vi "Measurement UI.vi"() -> ()   [LabVIEW 2021, in "Efficiency_Class D Amplifier_UI.lvlib"]
uses:
  Efficiency_Class D Amplifier_UI.lvlib
  shared/controls/units - snr.ctl
  shared/controls/units - ratio.ctl
  shared/controls/digital output level units.ctl
  shared/ui/controls/view.ctl
  shared/controls/power measurement method.ctl
  UI State.ctl
  <vilib>/Utility/miscctls.llb/LVBoundsTypeDef.ctl
  <vilib>/Utility/miscctls.llb/LVPoint32TypeDef.ctl
  shared/ui/UI Helpers.lvlib
  shared/controls/audio controls.lvlib
panel:
  in  "view legend":T1
  out "time domain":waveform(dbl)[](graph)
  out "frequency domain":cluster{"x0":dbl, "dx":dbl, "magnitude":dbl[]}[](graph)
  out "efficiency (%)":dbl caption="Efficiency" format="%#.2g%"
  out "power loss (W)":dbl caption="Power Loss" format="%#.2g W"
  out "total output power (W)":dbl caption="Total Output Power" format="%#.2g W"
  out "input power (W)":dbl caption="Input Power" format="%#.2g W"
  out "meas table":string[][](table)
  in  "power measurement resource":string="PXI1Slot4/ai0"
  out "output power (W)":dbl[](array[numeric])
  out "SFDR (dBc)":dbl[](array[numeric])
  out "gain":dbl[](array[numeric])
  out "dynamic range (dB)":dbl[](array[numeric])
  out "THD":dbl[](array[numeric])
  out "THD+N":dbl[](array[numeric])
  out "SNR":dbl[](array[numeric])
  out "phase (deg)":dbl[](array[numeric])
  out "amplitude (dBFS)":dbl[](array[numeric])
  out "amplitude (Vrms)":dbl[](array[numeric])
  out "frequency (Hz)":dbl[](array[numeric])
  out "channel names":string[](array[string])
  in  "Configuration tab":enum32{"Protocol", "Measurement", "Units"}(tab)
  in  "enable dither":bool caption="Enable dither"
  in  "master clock channel list":string caption="Master Clock Channel"
  in  "digital channel list":string caption="Digital Audio Channel"
  in  "logic level":enum32{"3.3 V", "1.8 V", "1.2 V"}(ring) caption="Logic level"
  in  "master clock rate":dbl=12288000.0 caption="Master clock rate" format="%#_6pHz"
  out "Bit clock rate":dbl=3072000.0 format="%#_6pHz"
  in  "number of channels":u32=2 caption="Number of channels"
  in  "TDM":bool
  in  "RJ":bool
  in  "LJ":bool
  in  "I2S":bool
  in  "bit clock edge sync":enum32{"Rising", "Falling"}(ring)=enum."Falling" caption="Bit clock edge sync"
  in  "frame clock rate":dbl=48000.0 caption="Frame clock rate" format="%#_6pHz"
  in  "data justification":enum32{"Left Justified", "Right Justified"}(ring) caption="Data justification"
  in  "endianness":enum32{"MSB First", "LSB First"}(ring) caption="Endianness"
  in  "bit depth":u32=24 caption="Bit depth"
  in  "channel length":u32=32 caption="Channel length"
  in  "frame sync edge for channel 0":enum32{"Rising", "Falling"}(ring)=enum."Falling" caption="Frame sync edge for Channel 0"
  in  "sense resistor (Ohms)":dbl caption="Sense Resistor" format="%#_g Ohms"
  in  "power supply current limit":dbl caption="Current Limit" format="%#_g A"
  in  "power supply voltage":dbl caption="Power Supply Voltage" format="%#_g V"
  in  "power meas resource":refnum<k15> caption="Resource"
  in  "power measurement method":T2 caption="Method"
  in  "output level":dbl=-1.0 caption="Output level" format="%#_3f"
  in  "output level units":T3
  in  "min settling cycles":u32 caption="Minimum settling cycles"
  in  "min settling time (s)":dbl=0.1 caption="Minimum settling time" format="%#_6ps"
  in  "min measurement cycles":u32 caption="Minimum measurement cycles"
  in  "min measurement time (s)":dbl=0.1 caption="Minimum measurement time" format="%#_6ps"
  in  "Acquisition channel":tag
  in  "acq sampling rate":dbl=51200.0 caption="Sample rate" format="%#.6pHz"
  in  "lowpass filter":T4(ring) caption="Lowpass filter"
  in  "highpass filter":enum32{"DC", "AC"}(ring) caption="Highpass filter"
  in  "band start":dbl=20.0 caption="Band start" format="%#_6pHz"
  in  "band stop":dbl=20000.0 caption="Band stop" format="%#_6pHz"
  in  "weighting filter":T5(ring)=enum."A-weighting" caption="Weighting filter"
  in  "load impedance":dbl=4.0 caption="Load impedance" format="%#_6p Ohms"
  in  "output range (pk-pk)":dbl=15.0 caption="Output range" format="%.3p Vpk-pk"
  in  "signal frequency":dbl=1000.0 caption="Frequency" format="%#_6pHz"
  in  "gain units":T6 caption="Gain"
  in  "THD units":T6 caption="THD"
  in  "THD+N units":T6 caption="THD+N"
  in  "SNR units":T7 caption="SNR"
  in  "channel 0 offset":u32=1
  out "fft - data":dbl[](array[numeric])
  out "fft - df":dbl
  out "fft - f0":dbl
  out "wfm - data":dbl[](array[numeric])
  out "wfm - dt":dbl
  out "wfm - t0":dbl
  in  "acq channel":string="PXI1Slot4/ai0"
  in  "signal phase":dbl caption="phase"
  # "hidden controls - used to sync with MeasLink"
  # "hidden indicators"
  # "Protocols"
  # "Audio Protocol"
  # "Clock Settings"
  # "Signal Level"
  # "Harware Resource"
  # "Filters"
  # "Output"
  # "Acquisition"
  # "Power"
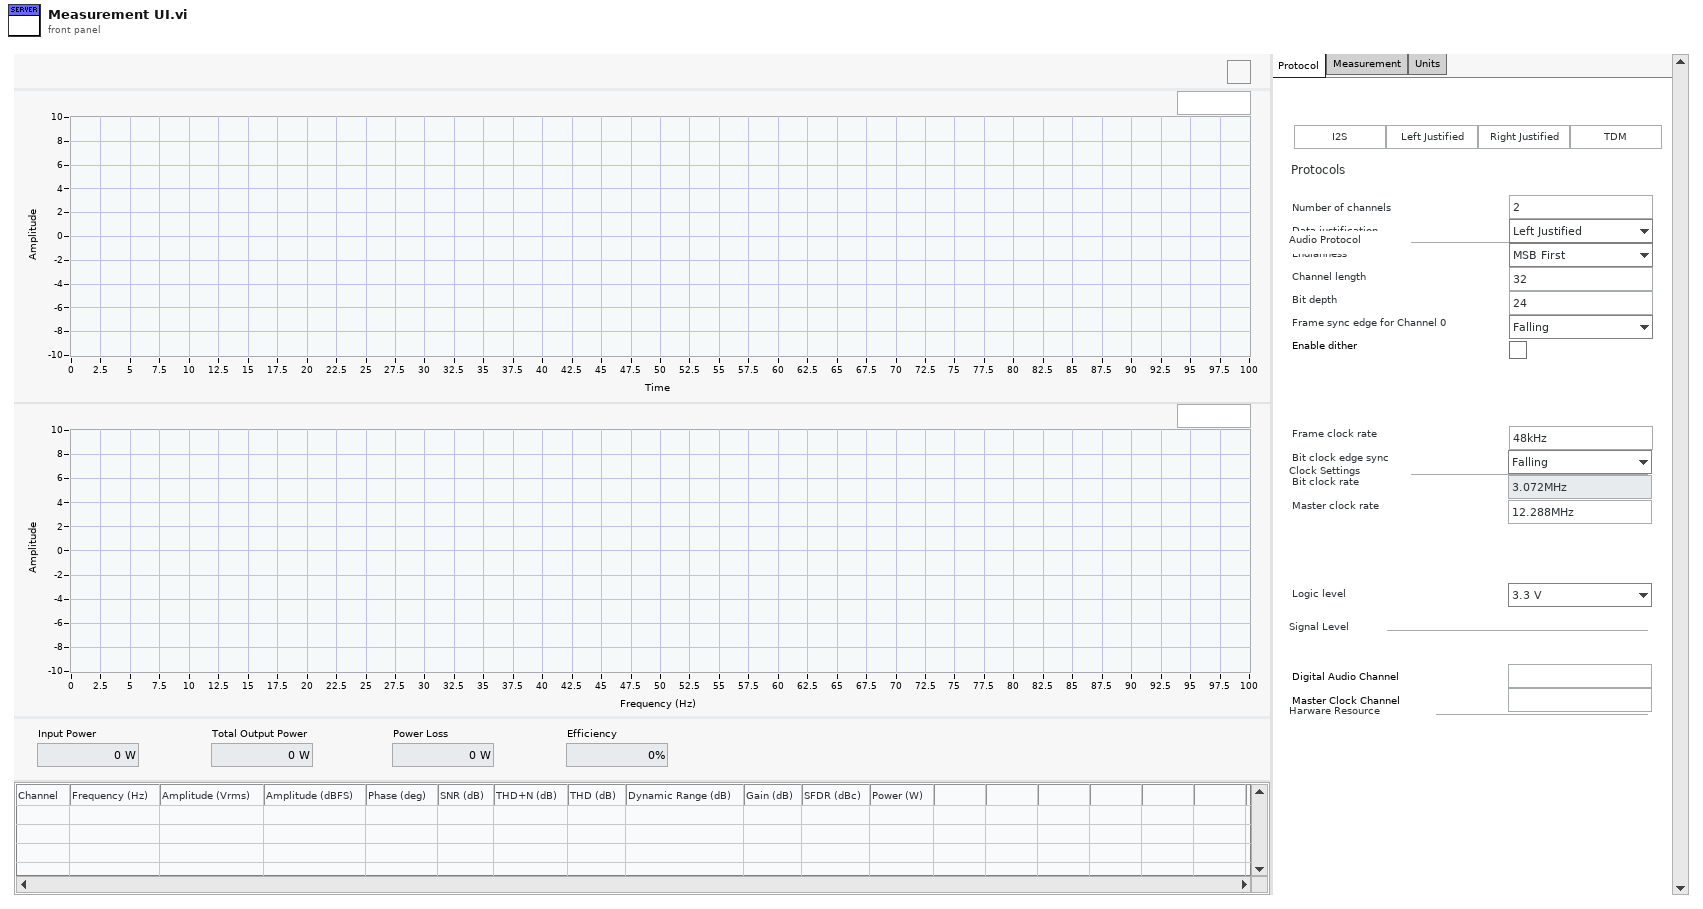
[diagram p1: front panel]
types:
  T1 = typedef "UI Helpers.lvlib/view.ctl" = bool
  T2 = typedef "power measurement method.ctl" = enum32{"SMU", "DMM"}
  T3 = typedef "audio controls.lvlib/digital output level units.ctl" = enum32{"% FS", "dBFS"}
  T4 = enum32{"No filter", "AES17 20kHz", "AES17 40kHz"}
  T5 = enum32{"Linear", "A-weighting", "B-weighting", "C-weighting"}
  T6 = typedef "audio controls.lvlib/units - ratio.ctl" = enum32{"dB", "%", "x/y"}
  T7 = typedef "audio controls.lvlib/units - snr.ctl" = enum32{"dB", "x/y"}
  T8 = typedef "Efficiency_Class D Amplifier_UI.lvlib/UI State.ctl" = cluster{"Graph Size":T9, "Legend Visible":bool, "Mouse Coords":T10}
  T9 = typedef "LVBoundsTypeDef.ctl" = cluster{"Width":u32, "Height":u32}
  T10 = typedef "LVPoint32TypeDef.ctl" = cluster{"Horizontal":i32, "Vertical":i32}
  T11 = typedef "LVPointTypeDef.ctl" = cluster{"Horizontal":i16, "Vertical":i16}
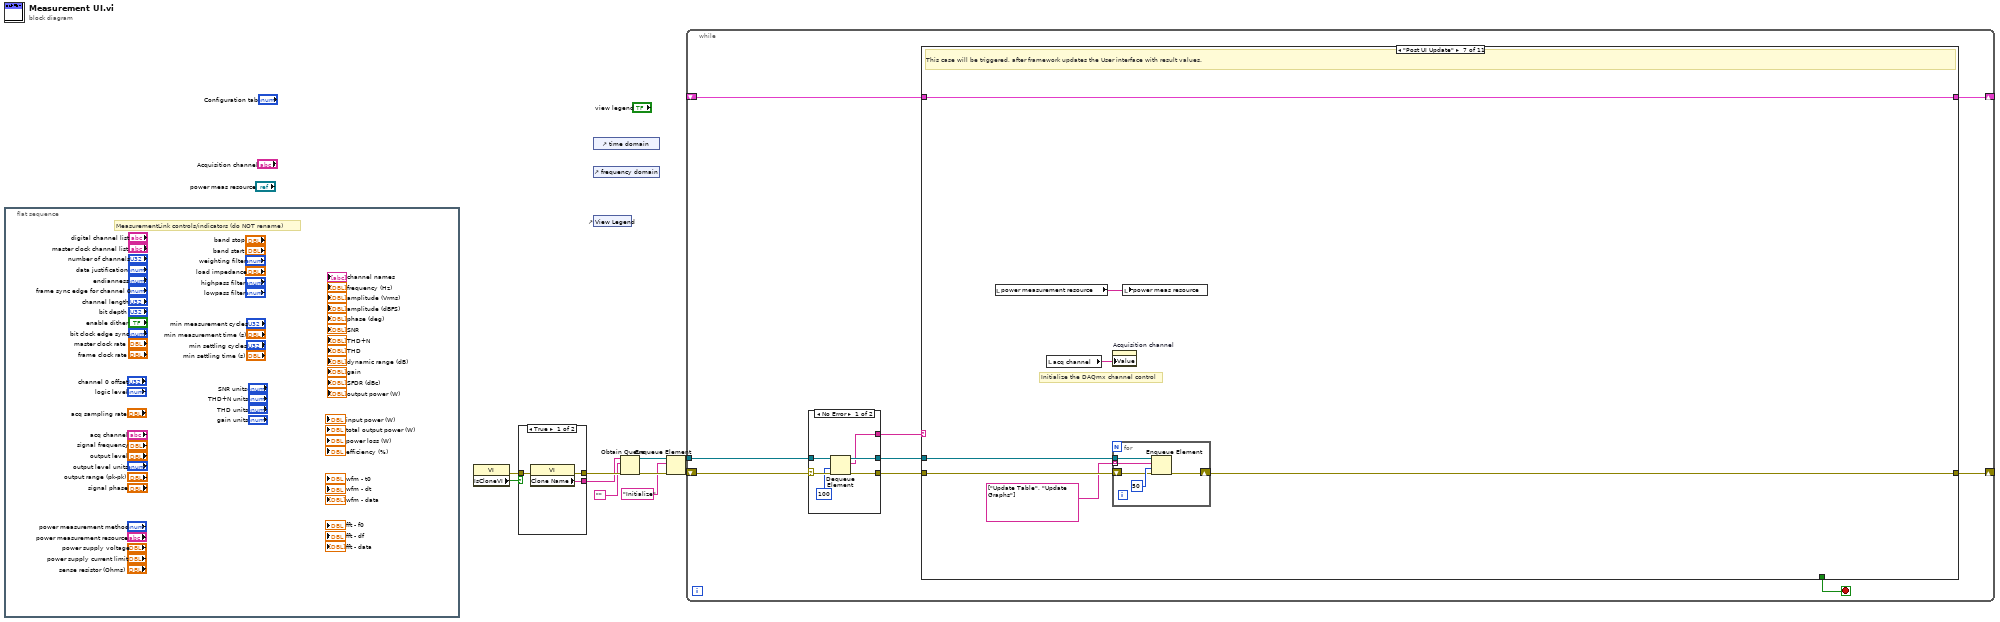
[diagram p0: block diagram]
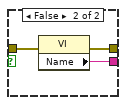
[diagram p2: hidden frame]
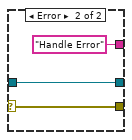
[diagram p3: hidden frame]
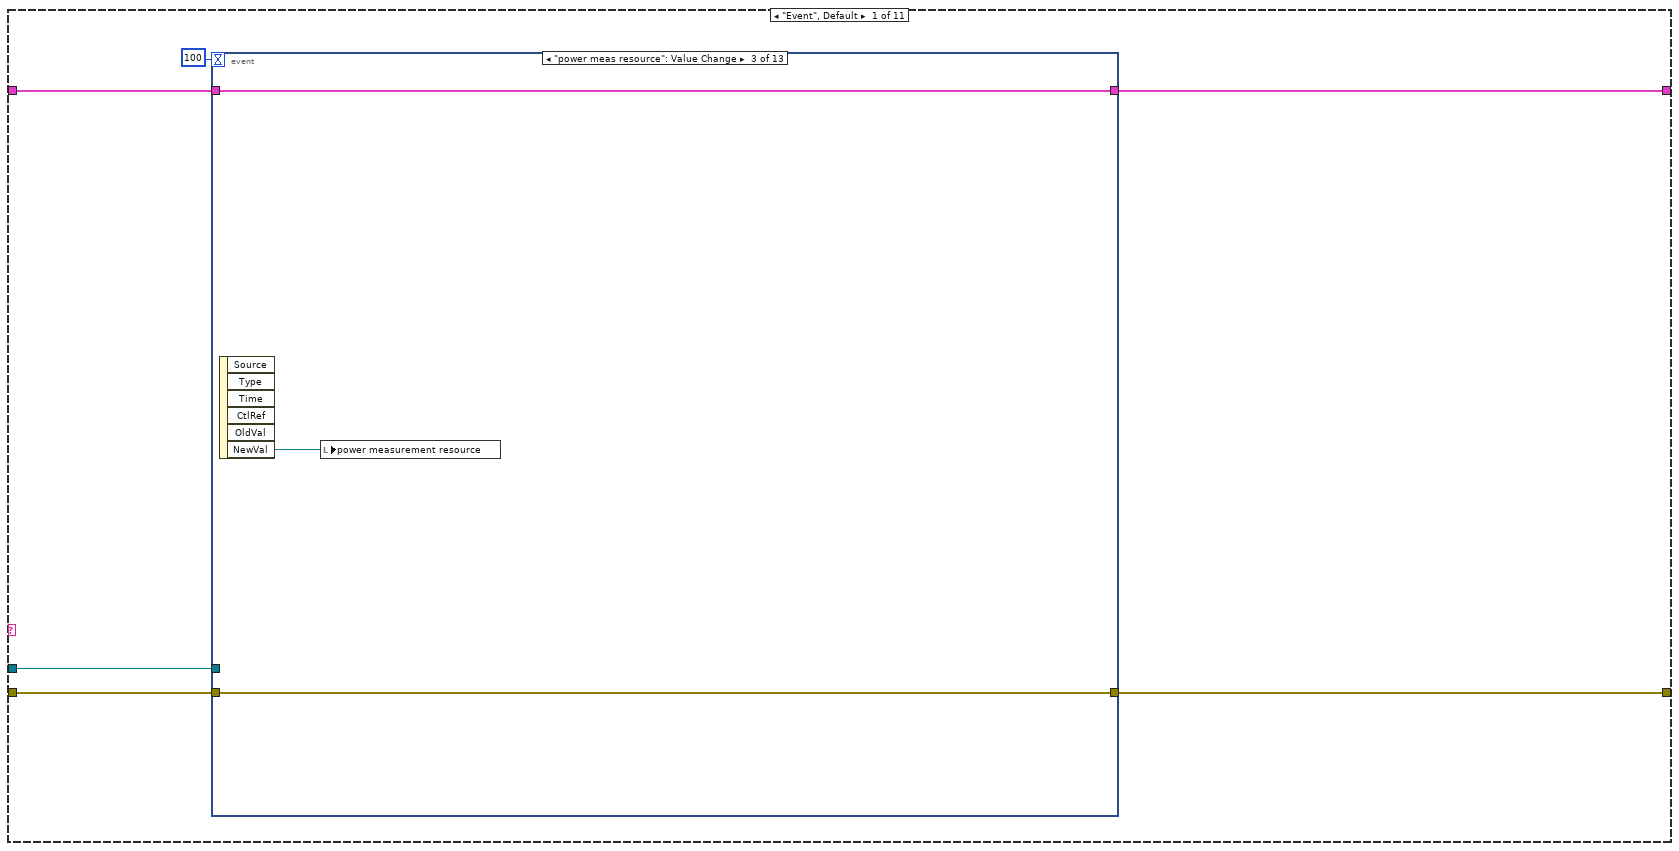
[diagram p4: hidden frame]
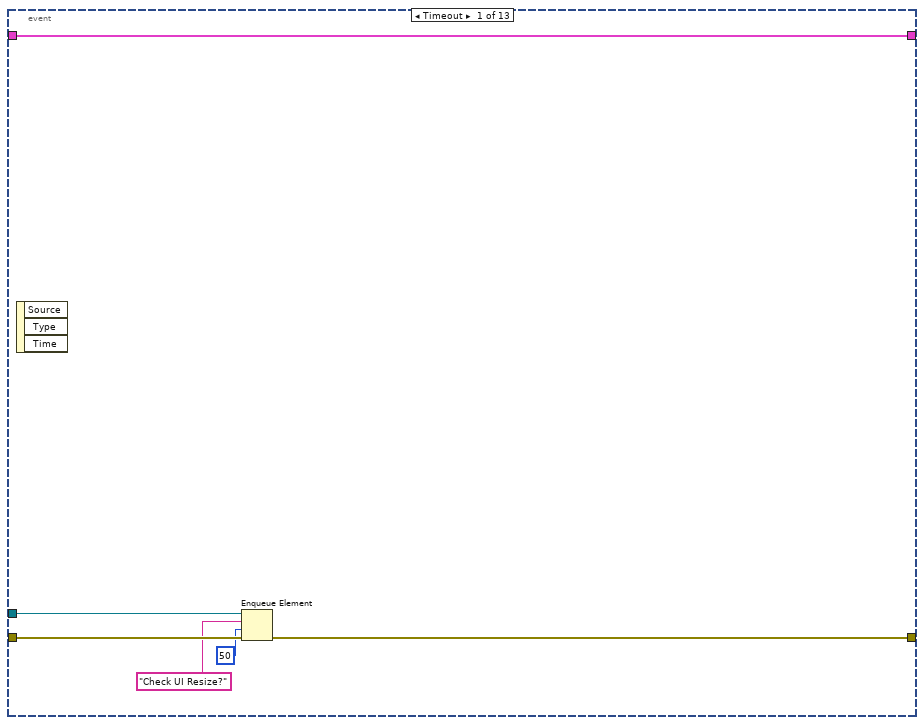
[diagram p5: hidden frame]
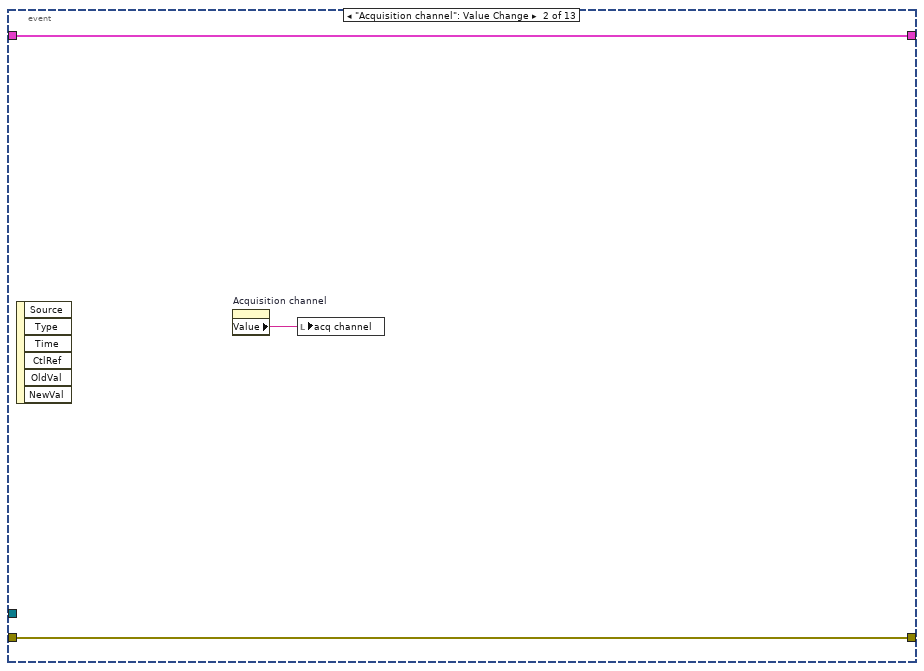
[diagram p6: hidden frame]
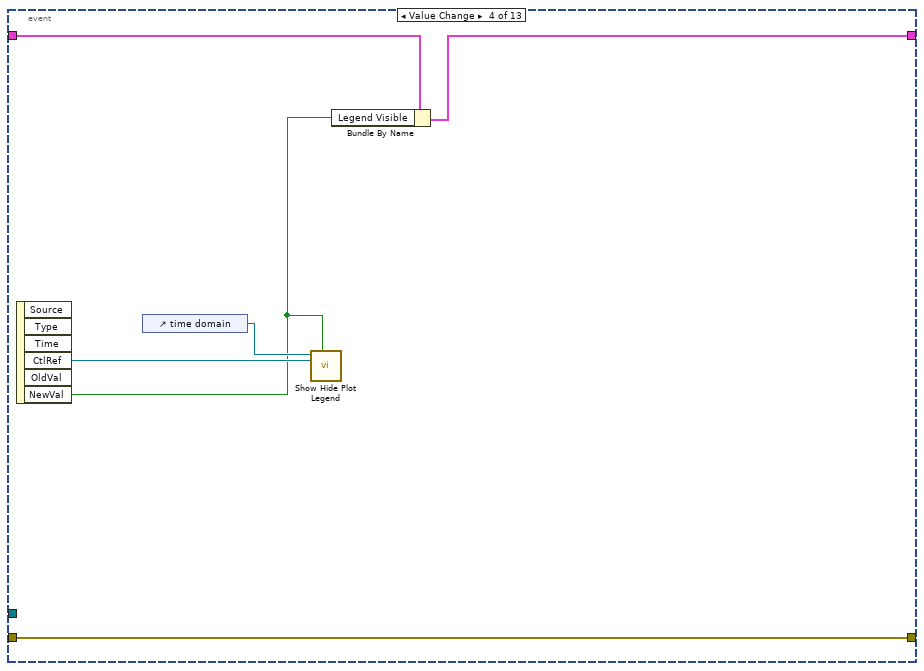
[diagram p7: hidden frame]
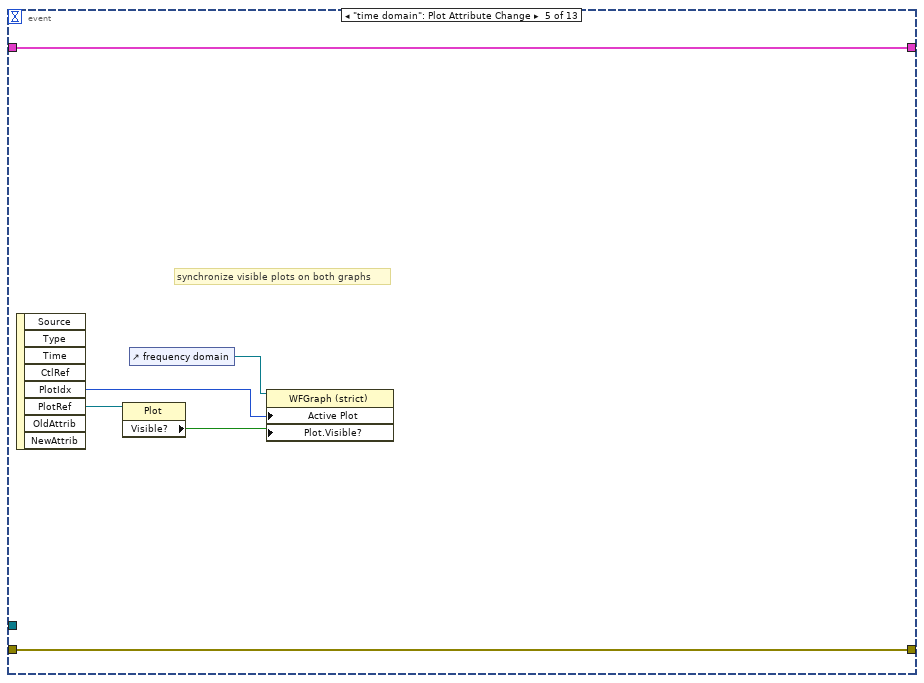
[diagram p8: hidden frame]
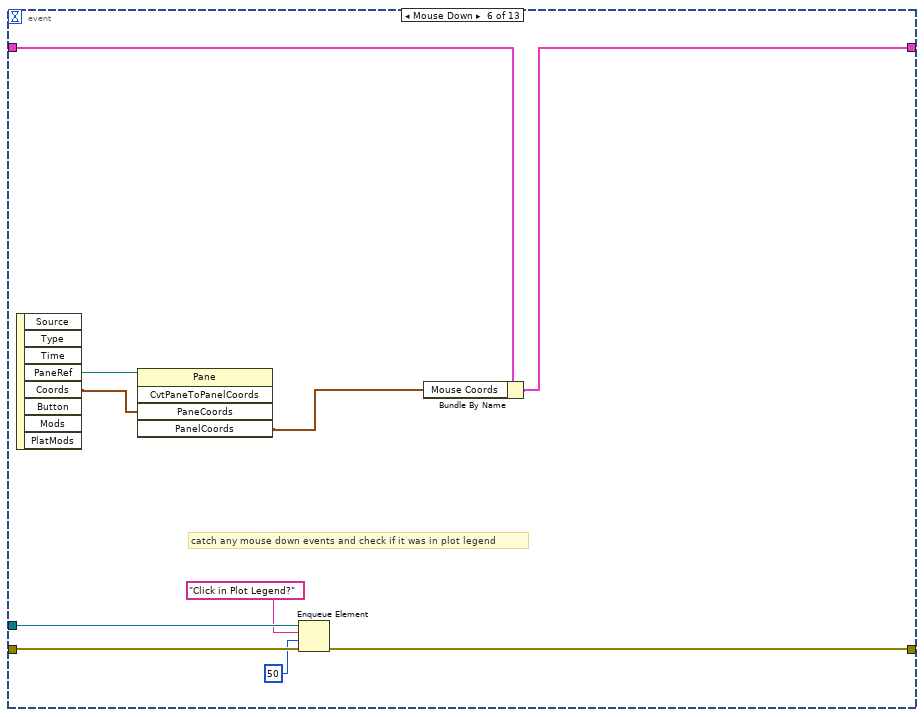
[diagram p9: hidden frame]
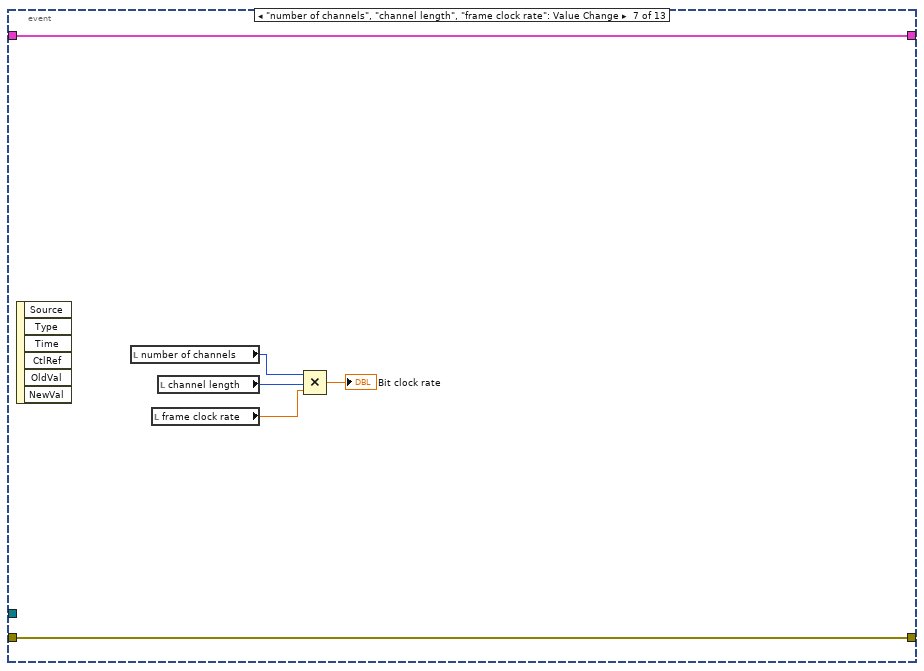
[diagram p10: hidden frame]
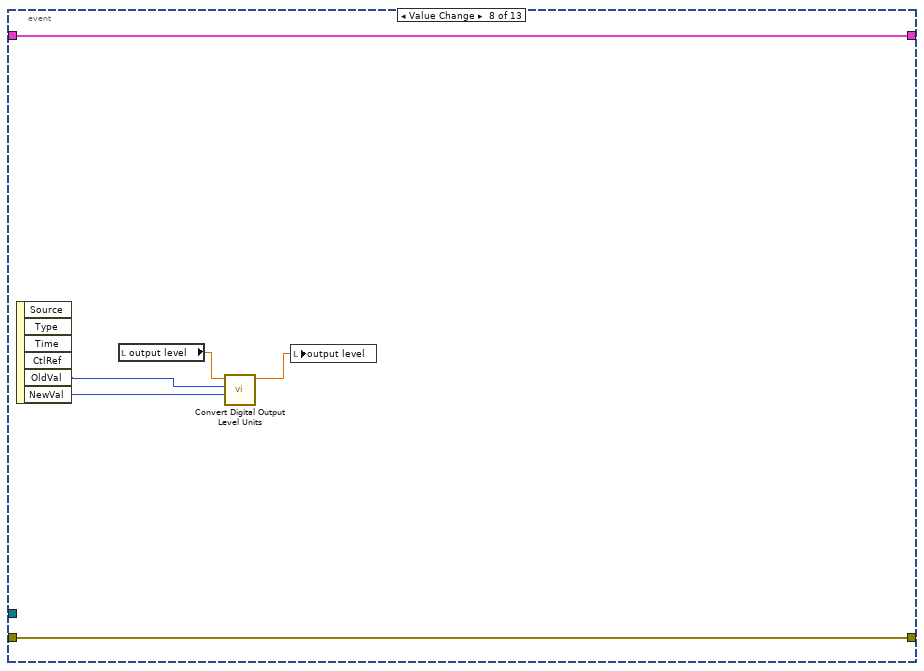
[diagram p11: hidden frame]
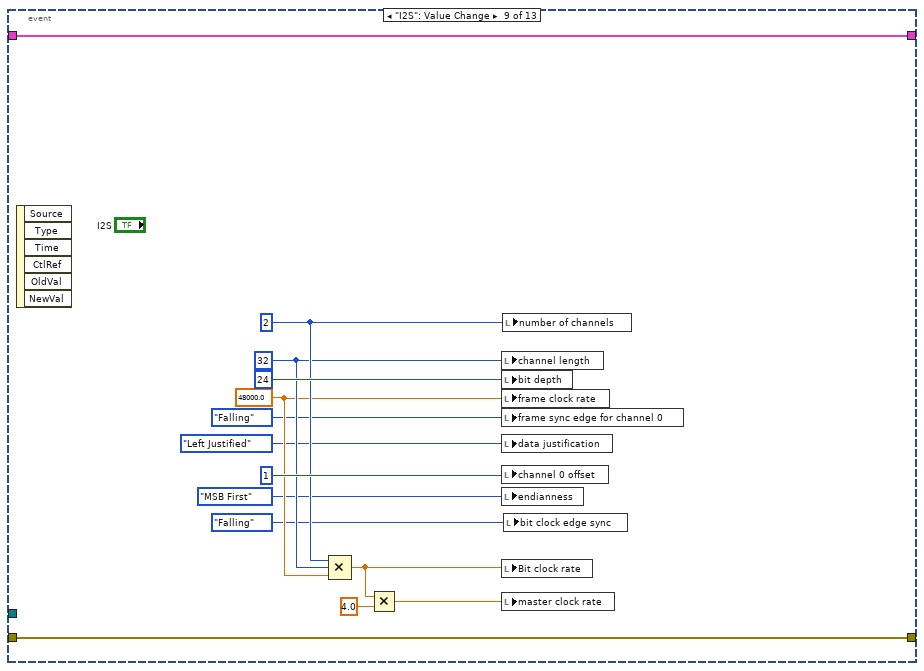
[diagram p12: hidden frame]
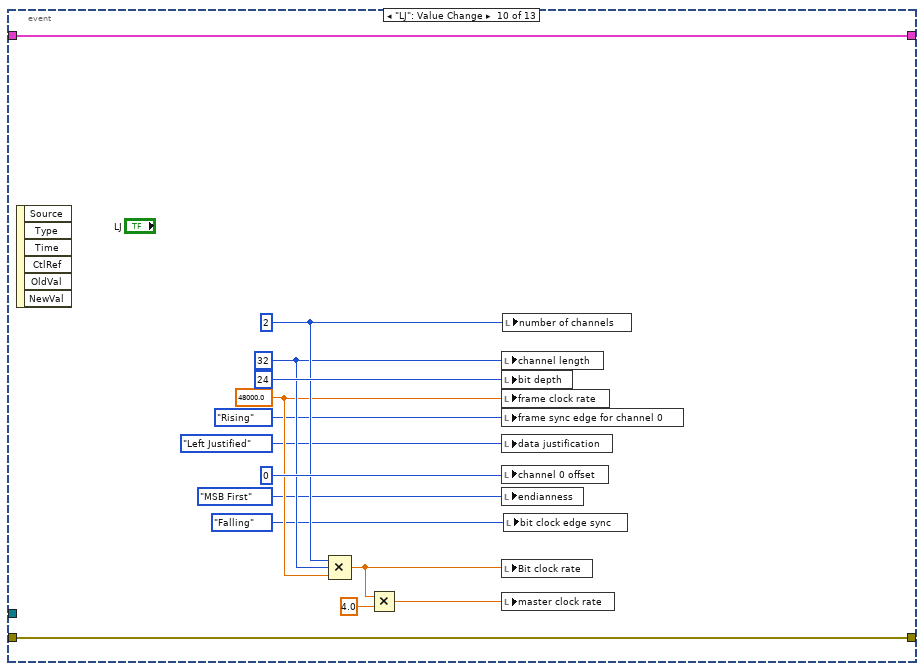
[diagram p13: hidden frame]
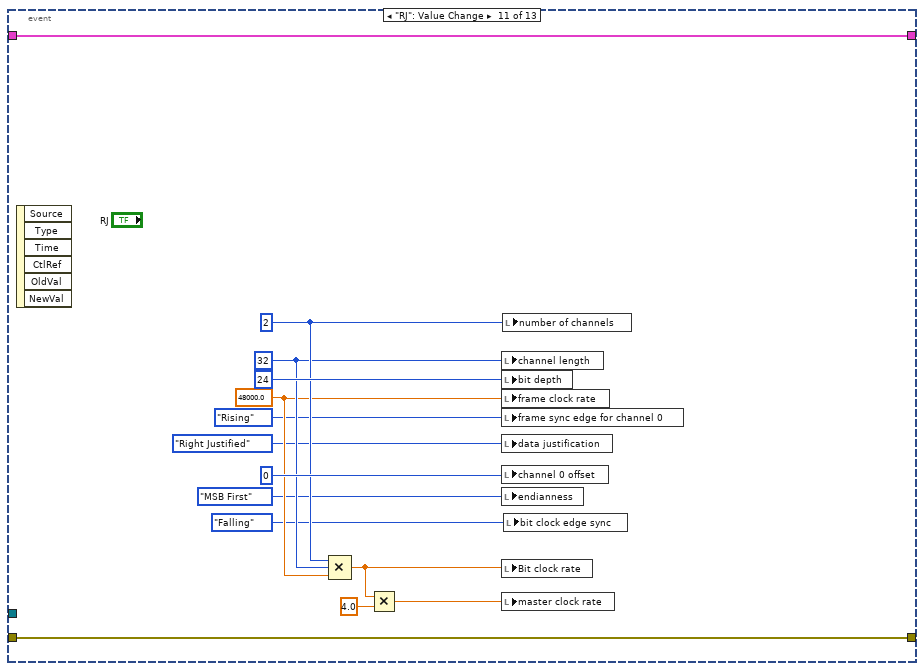
[diagram p14: hidden frame]
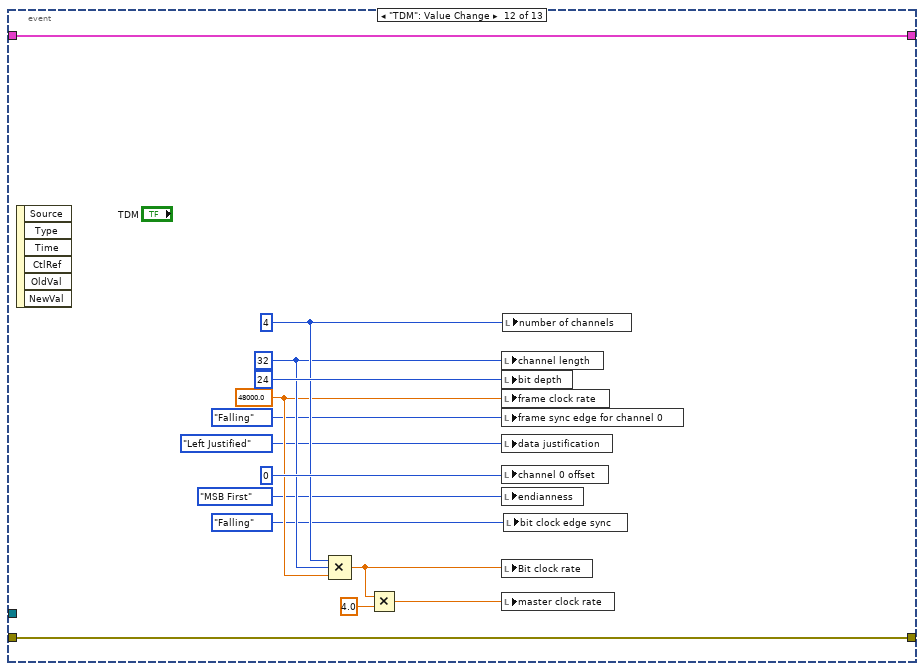
[diagram p15: hidden frame]
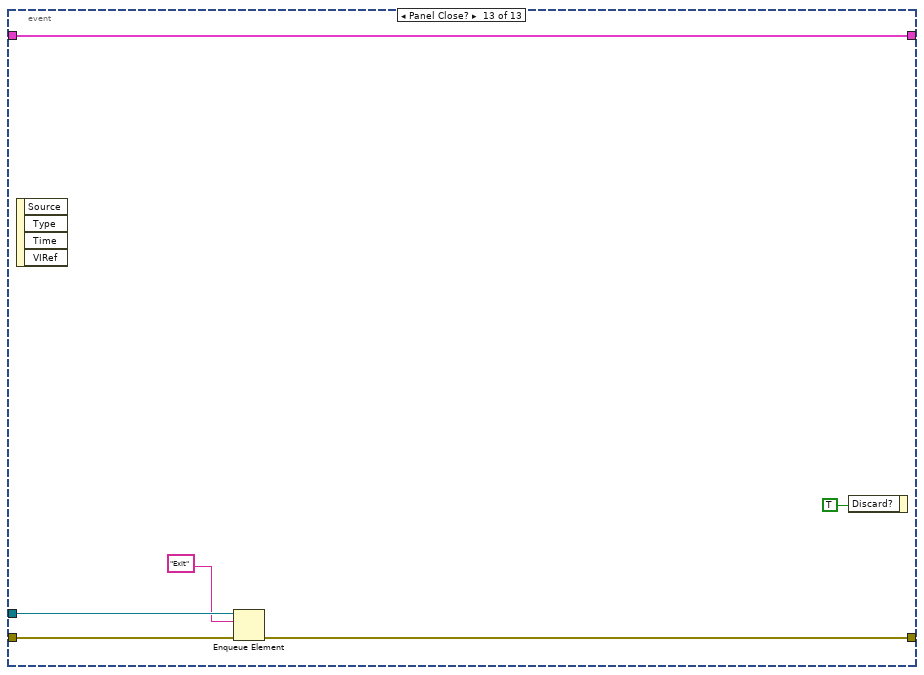
[diagram p16: hidden frame]
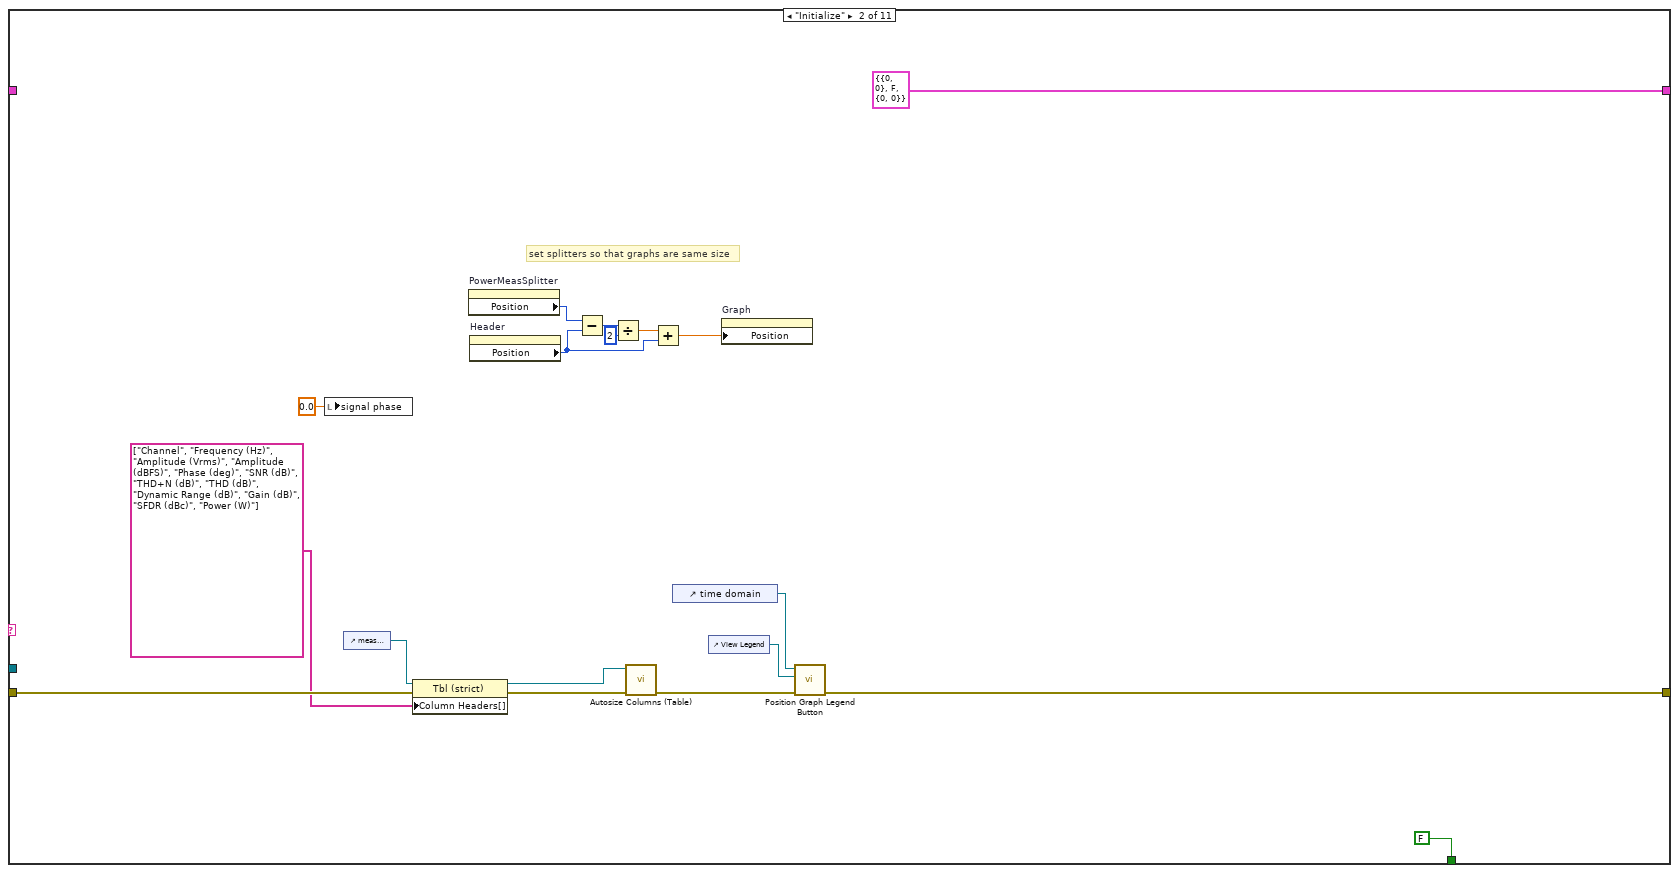
[diagram p17: hidden frame]
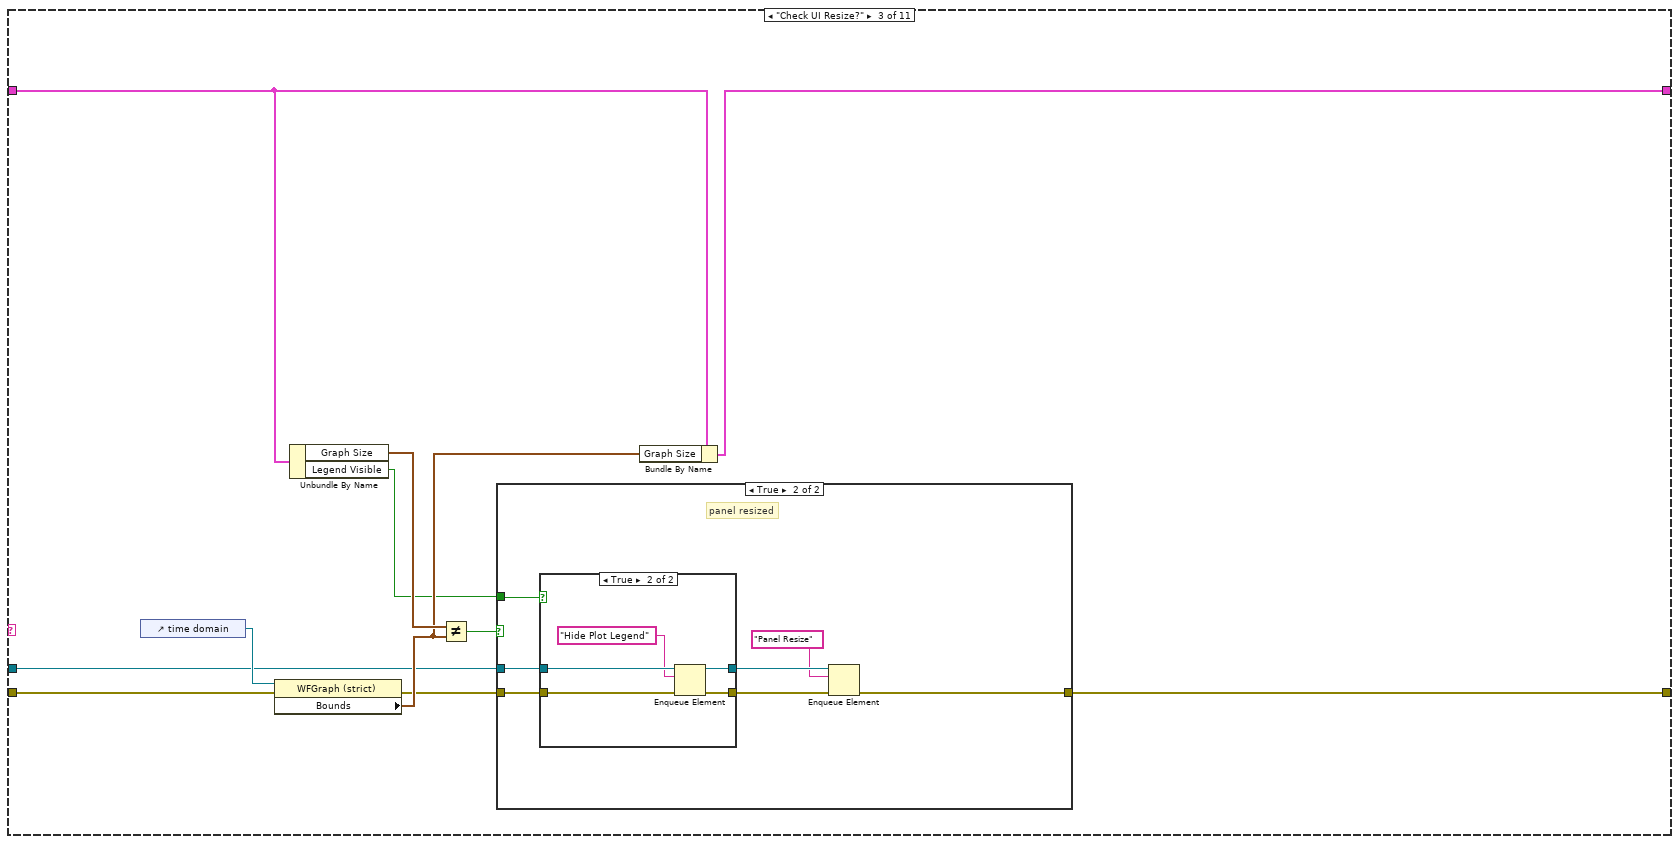
[diagram p18: hidden frame]
diagram:
  n1 = flat-sequence {
    frame #0 {
      # "MeasurementLink controls/indicators (do NOT rename)"
    }
  }
  n2 = property class="VI"() -> (error out=w1:errorcluster, "IsCloneVI"=w2:bool)  [unwired: 2 in, 1 out]
  n3 = case shown="True" w2 {
    tunnel: [w13 w16] -> w10
    tunnel: [w12 w15] -> w9
    tunnel: w1 -> [w11 w14]
    frame True {
      n4 = property class="VI"(error in=w11) -> (error out=w13:errorcluster, "Clone Name"=w12:string)  [unwired: 1 in, 1 out]
    }
    frame False {
      n5 = property class="VI"(error in=w14) -> (error out=w16:errorcluster, "Name"=w15:string)  [unwired: 1 in, 1 out]
    }
  }
  n6 = control-ref of="time domain"() -> ()  [unwired: 1 out]
  n7 = control-ref of="frequency domain"() -> ()  [unwired: 1 out]
  n8 = control-ref of="View Legend"() -> ()  [unwired: 1 out]
  n9 = Obtain Queue(name (unnamed)=w9, element data type="", error in (no error)=w10) -> (queue out=w6:refnum<queue>, error out=w8:errorcluster)  [unwired: 2 in, 1 out]
  n10 = Enqueue Element(queue=w6, element="Initialize", error in (no error)=w8) -> (queue out=w5:refnum<queue>, error out=w7:errorcluster)  [unwired: 1 in, 1 out]
  n11 = while {
    shift-right: [w20] -> _
    shift-left: w7 -> [w25]
    tunnel: w5 -> [w23]
    shift-right: [w18] -> _
    shift-left: _ -> [w17]
    stop <- w19 stop-if-true
    n12 = case shown="No Error" w25 {
      selector: w25 -> [w31 w34]
      tunnel: [w30 w34] -> w24
      tunnel: w23 -> [w29 w33]
      tunnel: [w28 w33] -> w22
      tunnel: [w27 "Handle Error"] -> w21
      frame No Error {
        n13 = Dequeue Element(queue=w29, timeout in ms (-1)=100, error in (no error)=w31) -> (queue out=w28:refnum<queue>, element=w27:string, error out=w30:errorcluster)  [unwired: 1 out]
      }
      frame Error {
      }
    }
    n14 = case shown="\"Post UI Update\"" w21 {
      tunnel: w24 -> [w39 w159 w176 w194 w216 w221 w229 w249 w257 w383 w385]
      tunnel: w22 -> [w37 _ w167 w195 _ _ w228 _ _ w381 _]
      tunnel: [w40 w160 w169 w193 w215 w220 w226 w249 w261 w378 w385] -> w20
      tunnel: [_ FALSE _ _ _ _ _ _ _ TRUE _] -> w19
      tunnel: [w35 T8 {"Graph Size"={"Width"=0, "Height"=0}, "Legend Visible"=FALSE, "Mouse Coords"={"Horizontal"=0, "Vertical"=0}} ("ui state") w172 w198 w217 w224 w230 w250 w258 w376 w384] -> w18
      tunnel: w17 -> [w36 _ w173 w198 w218 w224 w230 w250 w258 w376 w384]
      frame "Event", Default {
        n15 = event shown="[2] \"power meas resource\": Value Change" {
          selector: _ -> [_ _ _ _ _ _ _ _ _ _ _ _ _]
          dyn-events: _ -> [_ _ _ _ _ _ _ _ _ _ _ _ _]
          timeout: 100 -> [_ _ _ _ _ _ _ _ _ _ _ _ _]
          tunnel: [w43 w47 w52 w55 w59 w72 w75 w81 w87 w101 w115 w129 w146] -> w40
          tunnel: w39 -> [w46 w47 w52 w55 w59 w73 w75 w81 w87 w101 w115 w129 w147]
          tunnel: w37 -> [w45 _ _ _ _ w74 _ _ _ _ _ _ w145]
          tunnel: w36 -> [w42 w48 w51 w57 w60 w69 w76 w82 w88 w102 w116 w130 w143]
          tunnel: [w42 w48 w51 w56 w60 w68 w76 w82 w88 w102 w116 w130 w143] -> w35
          event Timeout {
            n16 = event-data() -> ()  [unwired: 1 in, 3 out]
            n17 = Enqueue Element(queue=w45, element="Check UI Resize?", timeout in ms (-1)=50, error in (no error)=w46) -> (error out=w43:errorcluster)  [unwired: 2 out]
          }
          event "Acquisition channel": Value Change {
            n18 = event-data() -> ()  [unwired: 1 in, 6 out]
            n19 = property on="Acquisition channel" class="DAQmxName"() -> ("Value"=w49:string)  [unwired: 2 in, 2 out]
            n20 = local write "acq channel"(w49) -> ()
          }
          event "power meas resource": Value Change {
            n21 = event-data() -> ("NewVal"=w50:refnum<k15>)  [unwired: 1 in, 5 out]
            n22 = local write "power measurement resource"(w50) -> ()
          }
          event Value Change {
            n23 = event-data() -> ("CtlRef"=w54:refnum<vi>, "NewVal"=w53:T1)  [unwired: 1 in, 4 out]
            n24 = control-ref of="time domain"() -> (w58:refnum<vi>)
            n25 = call "Show Hide Plot Legend.vi"("show"=w53, "view reference"=w54, "graph reference"=w58) -> ()  [unwired: 8 in, 1 out]
            n26 = Bundle By Name(cluster=w57, "Legend Visible"=w53) -> (w56:T8)
          }
          event "time domain": Plot Attribute Change {
            # "synchronize visible plots on both graphs"
            n27 = event-data() -> ("PlotIdx"=w62:i32, "PlotRef"=w63:refnum<vi>)  [unwired: 1 in, 6 out]
            n28 = property class="Plot"(reference=w63) -> ("Visible?"=w64:bool)  [unwired: 1 in, 2 out]
            n29 = control-ref of="frequency domain"() -> (w61:refnum<vi>)
            n30 = property on="Property Node" class="WFGraph (strict)"(reference=w61, "Active Plot"=w62, "Plot.Visible?"=w64) -> ()  [unwired: 1 in, 2 out]
          }
          event Mouse Down {
            # "catch any mouse down events and check if it was in plot legend"
            n31 = event-data() -> ("PaneRef"=w67:refnum<vi>, "Coords"=w66:T10)  [unwired: 1 in, 6 out]
            n32 = invoke class="Pane" method="CvtPaneToPanelCoords"(reference=w67, "PaneCoords"=w66) -> ("PanelCoords"=w65:T11)  [unwired: 3 in, 4 out]
            n33 = Enqueue Element(queue=w74, element="Click in Plot Legend?", timeout in ms (-1)=50, error in (no error)=w73) -> (error out=w72:errorcluster)  [unwired: 2 out]
            n34 = Bundle By Name(cluster=w69, "Mouse Coords"=w65) -> (w68:T8)
          }
          event "number of channels", "channel length", "frame clock rate": Value Change {
            n35 = event-data() -> ()  [unwired: 1 in, 6 out]
            n36 = local read "number of channels"() -> (w80:u32)
            n37 = local read "frame clock rate"() -> (w78:dbl)
            n38 = local read "channel length"() -> (w79:u32)
            n39 = Compound Arithmetic op=MULTIPLY(w80, w79, w78) -> (→"Bit clock rate":dbl)
          }
          event Value Change {
            n40 = event-data() -> ("OldVal"=w86:T3, "NewVal"=w85:T3)  [unwired: 1 in, 4 out]
            n41 = local read "output level"() -> (w84:dbl)
            n42 = call "Convert Digital Output Level Units.vi"("new output level units"=w85, "previous output level units"=w86, "previous output level"=w84) -> ("new output level"=w83:dbl)  [unwired: 8 in]
            n43 = local write "output level"(w83) -> ()
          }
          event "I2S": Value Change {
            w96 = 48000.0 ("Frame Clock Rate")
            w97 = u32 32 ("Channel Length")
            w98 = u32 2 ("Number of Channels")
            n44 = event-data() -> ()  [unwired: 1 in, 6 out]
            n45 = Compound Arithmetic op=MULTIPLY(w98, w97, w96) -> (w95:dbl)
            n46 = Multiply(x=w95, y=4.0) -> (x*y=w94:dbl)
            n47 = local write "channel length"(w97) -> ()
            n48 = local write "bit depth"(u32 24 ("Bit Depth")) -> ()
            n49 = local write "frame clock rate"(w96) -> ()
            n50 = local write "frame sync edge for channel 0"(enum32{"Rising", "Falling"}."Falling" ("bit clock edge sync")) -> ()
            n51 = local write "data justification"(enum32{"Left Justified", "Right Justified"}."Left Justified" ("data justification")) -> ()
            n52 = local write "channel 0 offset"(u32 1 ("Channel 0 Offset")) -> ()
            n53 = local write "endianness"(enum32{"MSB First", "LSB First"}."MSB First" ("endianness")) -> ()
            n54 = local write "Bit clock rate"(w95) -> ()
            n55 = local write "master clock rate"(w94) -> ()
            n56 = local write "number of channels"(w98) -> ()
            n57 = local write "bit clock edge sync"(enum32{"Rising", "Falling"}."Falling" ("frame sync edge for channel 0")) -> ()
          }
          event "LJ": Value Change {
            w110 = 48000.0 ("Frame Clock Rate")
            w111 = u32 32 ("Channel Length")
            w112 = u32 2 ("Number of Channels")
            n58 = event-data() -> ()  [unwired: 1 in, 6 out]
            n59 = Compound Arithmetic op=MULTIPLY(w112, w111, w110) -> (w109:dbl)
            n60 = Multiply(x=w109, y=4.0) -> (x*y=w108:dbl)
            n61 = local write "channel length"(w111) -> ()
            n62 = local write "bit depth"(u32 24 ("Bit Depth")) -> ()
            n63 = local write "frame clock rate"(w110) -> ()
            n64 = local write "frame sync edge for channel 0"(enum32{"Rising", "Falling"}."Rising" ("bit clock edge sync")) -> ()
            n65 = local write "data justification"(enum32{"Left Justified", "Right Justified"}."Left Justified" ("data justification")) -> ()
            n66 = local write "channel 0 offset"(u32 0 ("Channel 0 Offset")) -> ()
            n67 = local write "endianness"(enum32{"MSB First", "LSB First"}."MSB First" ("endianness")) -> ()
            n68 = local write "Bit clock rate"(w109) -> ()
            n69 = local write "master clock rate"(w108) -> ()
            n70 = local write "number of channels"(w112) -> ()
            n71 = local write "bit clock edge sync"(enum32{"Rising", "Falling"}."Falling" ("frame sync edge for channel 0")) -> ()
          }
          event "RJ": Value Change {
            w124 = 48000.0 ("Frame Clock Rate")
            w125 = u32 32 ("Channel Length")
            w126 = u32 2 ("Number of Channels")
            n72 = event-data() -> ()  [unwired: 1 in, 6 out]
            n73 = Compound Arithmetic op=MULTIPLY(w126, w125, w124) -> (w123:dbl)
            n74 = Multiply(x=w123, y=4.0) -> (x*y=w122:dbl)
            n75 = local write "channel length"(w125) -> ()
            n76 = local write "bit depth"(u32 24 ("Bit Depth")) -> ()
            n77 = local write "frame clock rate"(w124) -> ()
            n78 = local write "frame sync edge for channel 0"(enum32{"Rising", "Falling"}."Rising" ("bit clock edge sync")) -> ()
            n79 = local write "data justification"(enum32{"Left Justified", "Right Justified"}."Right Justified" ("data justification")) -> ()
            n80 = local write "channel 0 offset"(u32 0 ("Channel 0 Offset")) -> ()
            n81 = local write "endianness"(enum32{"MSB First", "LSB First"}."MSB First" ("endianness")) -> ()
            n82 = local write "Bit clock rate"(w123) -> ()
            n83 = local write "master clock rate"(w122) -> ()
            n84 = local write "number of channels"(w126) -> ()
            n85 = local write "bit clock edge sync"(enum32{"Rising", "Falling"}."Falling" ("frame sync edge for channel 0")) -> ()
          }
          event "TDM": Value Change {
            w138 = 48000.0 ("Frame Clock Rate")
            w139 = u32 32 ("Channel Length")
            w140 = u32 4 ("Number of Channels")
            n86 = event-data() -> ()  [unwired: 1 in, 6 out]
            n87 = Compound Arithmetic op=MULTIPLY(w140, w139, w138) -> (w137:dbl)
            n88 = Multiply(x=w137, y=4.0) -> (x*y=w136:dbl)
            n89 = local write "channel length"(w139) -> ()
            n90 = local write "bit depth"(u32 24 ("Bit Depth")) -> ()
            n91 = local write "frame clock rate"(w138) -> ()
            n92 = local write "frame sync edge for channel 0"(enum32{"Rising", "Falling"}."Falling" ("bit clock edge sync")) -> ()
            n93 = local write "data justification"(enum32{"Left Justified", "Right Justified"}."Left Justified" ("data justification")) -> ()
            n94 = local write "channel 0 offset"(u32 0 ("Channel 0 Offset")) -> ()
            n95 = local write "endianness"(enum32{"MSB First", "LSB First"}."MSB First" ("endianness")) -> ()
            n96 = local write "Bit clock rate"(w137) -> ()
            n97 = local write "master clock rate"(w136) -> ()
            n98 = local write "number of channels"(w140) -> ()
            n99 = local write "bit clock edge sync"(enum32{"Rising", "Falling"}."Falling" ("frame sync edge for channel 0")) -> ()
          }
          event Panel Close? {
            n100 = event-data() -> ()  [unwired: 1 in, 4 out]
            n101 = Enqueue Element(queue=w145, element="Exit", error in (no error)=w147) -> (error out=w146:errorcluster)  [unwired: 1 in, 2 out]
            n102 = event-data("Discard?"=TRUE) -> ()  [unwired: 1 in, 1 out]
          }
        }
      }
      frame "Initialize" {
        # "set splitters so that graphs are same size"
        n103 = local write "signal phase"(0.0 ("signal phase")) -> ()
        n104 = control-ref of="meas table"() -> (w157:refnum<vi>)
        n105 = property class="Tbl (strict)"(reference=w157, error in=w159, "Column Headers[]"=string[] ["Channel", "Frequency (Hz)", "Amplitude (Vrms)", "Amplitude (dBFS)", "Phase (deg)", "SNR (dB)", "THD+N (dB)", "THD (dB)", "Dynamic Range (dB)", "Gain (dB)", "SFDR (dBc)", "Power (W)"] ("Column Header Strings[]")) -> (reference out=w156:refnum<vi>, error out=w158:errorcluster)
        n106 = property on="PowerMeasSplitter" class="Splitter"() -> ("Position"=w154:i32)  [unwired: 2 in, 2 out]
        n107 = property on="Header" class="Splitter"() -> ("Position"=w150:i32)  [unwired: 2 in, 2 out]
        n108 = Subtract(x=w154, y=w150) -> (x-y=w153:i32)
        n109 = Divide(x=w153, y=2) -> (x/y=w151:dbl)
        n110 = call "Autosize Columns (Table).vi"("error in (no error)"=w158, "table"=w156) -> ("error out"=w161:errorcluster)  [unwired: 9 in]
        n111 = Add(x=w151, y=w150) -> (x+y=w149:dbl)
        n112 = control-ref of="time domain"() -> (w164:refnum<vi>)
        n113 = control-ref of="View Legend"() -> (w163:refnum<vi>)
        n114 = property on="Graph" class="Splitter"("Position"=w149) -> ()  [unwired: 2 in, 2 out]
        n115 = call "Position Graph Legend Button.vi"("error in (no error)"=w161, "view legend"=w163, "graph"=w164) -> ("error out"=w160:errorcluster)  [unwired: 8 in]
      }
      frame "Check UI Resize?" {
        n116 = control-ref of="time domain"() -> (w177:refnum<vi>)
        n117 = property on="Property Node" class="WFGraph (strict)"(reference=w177, error in=w176) -> (error out=w170:errorcluster, "Bounds"=w174:T9)  [unwired: 1 out]
        n118 = Unbundle By Name(w173) -> ("Graph Size"=w175:T9, "Legend Visible"=w168:bool)
        n119 = Not Equal?(x=w175, y=w174) -> (x != y?=w171:bool)
        n120 = case shown="True" w171 {
          tunnel: w170 -> [w178 w185]
          tunnel: [w178 w180] -> w169
          tunnel: w168 -> [_ w183]
          tunnel: w167 -> [_ w184]
          frame False {
            # "no resize"
          }
          frame True {
            # "panel resized"
            n121 = case shown="True" w183 {
              tunnel: w185 -> [w187 w192]
              tunnel: [w187 w191] -> w182
              tunnel: w184 -> [w186 w190]
              tunnel: [w186 w188] -> w181
              frame False {
              }
              frame True {
                n122 = Enqueue Element(queue=w190, element="Hide Plot Legend", error in (no error)=w192) -> (queue out=w188:refnum<queue>, error out=w191:errorcluster)  [unwired: 1 in, 1 out]
              }
            }
            n123 = Enqueue Element(queue=w181, element="Panel Resize", error in (no error)=w182) -> (error out=w180:errorcluster)  [unwired: 1 in, 2 out]
          }
        }
        n124 = Bundle By Name(cluster=w173, "Graph Size"=w174) -> (w172:T8)
      }
      frame "Click in Plot Legend?" {
        n125 = Unbundle By Name(w198) -> ("Legend Visible"=w197:bool, "Mouse Coords"=w196:T10)
        n126 = case shown="True" w197 {
          tunnel: w196 -> [_ w204]
          tunnel: w195 -> [_ w201]
          tunnel: w194 -> [w199 w206]
          tunnel: [w199 w200] -> w193
          frame False {
            # "legend not visible; do nothing"
          }
          frame True {
            # "check if mouse down in legend"
            n127 = control-ref of="time domain"() -> (w205:refnum<vi>)
            n128 = call "Check if Click in Graph Legend.vi"("error in (no error)"=w206, "Mouse Coords"=w204, "WaveformGraph"=w205) -> ("error out"=w202:errorcluster, "click in legend?"=w203:bool)  [unwired: 7 in]
            n129 = case shown="False" w203 {
              tunnel: w202 -> [w210 w211]
              tunnel: w201 -> [w209 _]
              tunnel: [w208 w211] -> w200
              frame False {
                n130 = Enqueue Element(queue=w209, element="Hide Plot Legend", error in (no error)=w210) -> (error out=w208:errorcluster)  [unwired: 1 in, 2 out]
              }
              frame True {
                # "inside legend; do nothing"
              }
            }
          }
        }
      }
      frame "Hide Plot Legend" {
        n131 = control-ref of="time domain"() -> (w213:refnum<vi>)
        n132 = control-ref of="View Legend"() -> (w212:refnum<vi>)
        n133 = call "Show Hide Plot Legend.vi"("show"=FALSE, "error in (no error)"=w216, "view reference"=w212, "graph reference"=w213) -> ("error out"=w215:errorcluster)  [unwired: 7 in]
        n134 = Bundle By Name(cluster=w218, "Legend Visible"=FALSE ("legend visible")) -> (w217:T8)
      }
      frame "Panel Resize" {
        n135 = control-ref of="time domain"() -> (w223:refnum<vi>)
        n136 = control-ref of="View Legend"() -> (w222:refnum<vi>)
        n137 = call "Position Graph Legend Button.vi"("error in (no error)"=w221, "view legend"=w222, "graph"=w223) -> ("error out"=w220:errorcluster)  [unwired: 8 in]
      }
      frame "Post UI Update" {
        # "Initialize the DAQmx channel control"
        # "This case will be triggered, after framework updates the User interface with result values."
        n138 = local read "power measurement resource"() -> (w225:string)
        n139 = local read "acq channel"() -> (w231:string)
        n140 = for {
          tunnel: w228 -> [w234]
          shift-right: [w233] -> w226
          shift-left: w229 -> [w235]
          tunnel: string[] ["Update Table", "Update Graphs"] -> [w232] mode=indexing
          n141 = Enqueue Element(queue=w234, element=w232, timeout in ms (-1)=50, error in (no error)=w235) -> (error out=w233:errorcluster)  [unwired: 2 out]
        }
        n142 = property on="Acquisition channel" class="DAQmxName"("Value"=w231) -> ()  [unwired: 2 in, 2 out]
        n143 = local write "power meas resource"(w225) -> ()
      }
      frame "Update Graphs" {
        # "This case will be triggered, after framework updates the User interface with result values."
        n144 = local read "channel names"() -> (w238:string[])
        n145 = control-ref of="time domain"() -> (w241:refnum<vi>)
        n146 = control-ref of="frequency domain"() -> (w237:refnum<vi>)
        n147 = local read "wfm - data"() -> (w248:dbl[])
        n148 = local read "wfm - dt"() -> (w247:dbl)
        n149 = local read "fft - data"() -> (w245:dbl[])
        n150 = local read "fft - df"() -> (w244:dbl)
        n151 = local read "fft - f0"() -> (w243:dbl)
        n152 = call "Array to Wfm (N Ch).vi"("channel names"=w238, "dt"=w247, "array"=w248) -> ("waveforms"=→"time domain":waveform(dbl)[])  [unwired: 8 in]
        n153 = call "Array to Spectrum (N Ch).vi"("channel names"=w238, "f0"=w243, "df"=w244, "array"=w245) -> ("spectra"=→"frequency domain":cluster{"x0":dbl, "dx":dbl, "magnitude":dbl[]}[])  [unwired: 7 in]
        n154 = for {
          tunnel: w237 -> [w251]
          tunnel: w238 -> [_] mode=indexing
          i -> [w252]
          # "make all plots visible"
          n155 = property class="WFGraph (strict)"(reference=w251, "Active Plot"=w252, "Plot.Visible?"=TRUE ("Plot.Visible")) -> ()  [unwired: 1 in, 2 out]
        }
        n156 = for {
          tunnel: w241 -> [w254]
          tunnel: w238 -> [_] mode=indexing
          i -> [w255]
          # "make all plots visible"
          n157 = property class="WFGraph (strict)"(reference=w254, "Active Plot"=w255, "Plot.Visible?"=TRUE ("Plot.Visible")) -> ()  [unwired: 1 in, 2 out]
        }
        n158 = Array Size(array=w238) -> (size(s)=w240:i32)
        n159 = property class="WFGraph (strict)"(reference=w241, "LegNumRows"=w240, "LegScrollVis"=FALSE ("Legend:Scrollbar Visible")) -> ()  [unwired: 1 in, 2 out]
      }
      frame "Update Table" {
        # "format data for table"
        # "This case will be triggered, after framework updates the User interface with result values."
        n160 = local read "SNR units"() -> (w301:T7)
        n161 = local read "THD+N units"() -> (w313:T6)
        n162 = local read "THD units"() -> (w299:T6)
        n163 = local read "gain units"() -> (w297:T6)
        n164 = case shown="\"x/y\"" w301 {
          tunnel: ["(dB)" "(ratio)"] -> w312
          tunnel: ["%5.1f" ("initial string") "%.1f" ("initial string")] -> w295
          frame "dB", Default {
          }
          frame "x/y" {
          }
        }
        n165 = case shown="\"x/y\"" w313 {
          tunnel: ["(dB)" "(%)" "(ratio)"] -> w315
          tunnel: ["%5.1f" ("initial string") "%.3f" ("initial string") "%.6f" ("initial string")] -> w292
          frame "dB", Default {
          }
          frame "%" {
          }
          frame "x/y" {
          }
        }
        n166 = case shown="\"x/y\"" w299 {
          tunnel: ["(dB)" "(%)" "(ratio)"] -> w300
          tunnel: ["%5.1f" ("initial string") "%.3f" ("initial string") "%.6f" ("initial string")] -> w289
          frame "dB", Default {
          }
          frame "%" {
          }
          frame "x/y" {
          }
        }
        n167 = case shown="\"%\"" w297 {
          tunnel: ["(dB)" "(%)" "(ratio)"] -> w298
          tunnel: ["%5.1f" ("initial string") "%.1f" ("initial string") "%.3f" ("initial string")] -> w279
          frame "dB", Default {
          }
          frame "%" {
          }
          frame "x/y" {
          }
        }
        n168 = Concatenate Strings("SNR " ("string"), w312) -> (w309:string)
        n169 = Concatenate Strings("THD+N " ("string"), w315) -> (w308:string)
        n170 = Concatenate Strings("Gain " ("string"), w298) -> (w306:string)
        n171 = Concatenate Strings("THD " ("string"), w300) -> (w307:string)
        n172 = property on="meas table" class="Tbl (strict)"() -> ("Column Headers[]"=w262:string[])  [unwired: 2 in, 2 out]
        n173 = Replace Array Subset(array=w262, new element #1=w309, index #1=5 ("index"), new element #2=w308, index #2=6 ("index"), new element #3=w307, index #3=7 ("index"), new element #4=w306, index #4=9 ("index")) -> (w310:string[])
        n174 = property on="meas table" class="Tbl (strict)"("Column Headers[]"=w310) -> ()  [unwired: 2 in, 2 out]
        n175 = local read "amplitude (Vrms)"() -> (w274:dbl[])
        n176 = local read "amplitude (dBFS)"() -> (w271:dbl[])
        n177 = local read "frequency (Hz)"() -> (w277:dbl[])
        n178 = local read "phase (deg)"() -> (w267:dbl[])
        n179 = local read "THD+N"() -> (w294:dbl[])
        n180 = local read "THD"() -> (w291:dbl[])
        n181 = local read "SNR"() -> (w296:dbl[])
        n182 = local read "channel names"() -> (w259:string[])
        n183 = for {
          tunnel: [w332] -> w276 mode=indexing
          tunnel: w277 -> [w331] mode=indexing
          tunnel: "%.3f" ("initial string") -> [w330]
          n184 = Format Into String(format string=w330, w331) -> (resulting string=w332:string)  [unwired: 2 in, 1 out]
        }
        n185 = for {
          tunnel: [w329] -> w273 mode=indexing
          tunnel: w274 -> [w328] mode=indexing
          tunnel: "%.3f" ("initial string") -> [w327]
          n186 = Format Into String(format string=w327, w328) -> (resulting string=w329:string)  [unwired: 2 in, 1 out]
        }
        n187 = for {
          tunnel: [w326] -> w270 mode=indexing
          tunnel: w271 -> [w325] mode=indexing
          tunnel: "%.3f" ("initial string") -> [w324]
          n188 = Format Into String(format string=w324, w325) -> (resulting string=w326:string)  [unwired: 2 in, 1 out]
        }
        n189 = for {
          tunnel: [w347] -> w290 mode=indexing
          tunnel: w291 -> [w346] mode=indexing
          tunnel: w289 -> [w345]
          n190 = Format Into String(format string=w345, w346) -> (resulting string=w347:string)  [unwired: 2 in, 1 out]
        }
        n191 = for {
          tunnel: [w353] -> w285 mode=indexing
          tunnel: w296 -> [w352] mode=indexing
          tunnel: w295 -> [w351]
          n192 = Format Into String(format string=w351, w352) -> (resulting string=w353:string)  [unwired: 2 in, 1 out]
        }
        n193 = for {
          tunnel: [w350] -> w293 mode=indexing
          tunnel: w294 -> [w349] mode=indexing
          tunnel: w292 -> [w348]
          n194 = Format Into String(format string=w348, w349) -> (resulting string=w350:string)  [unwired: 2 in, 1 out]
        }
        n195 = for {
          tunnel: [w323] -> w268 mode=indexing
          tunnel: w267 -> [w322] mode=indexing
          tunnel: "%.3f" ("initial string") -> [w321]
          n196 = Format Into String(format string=w321, w322) -> (resulting string=w323:string)  [unwired: 2 in, 1 out]
        }
        n197 = local read "dynamic range (dB)"() -> (w287:dbl[])
        n198 = local read "output power (W)"() -> (w283:dbl[])
        n199 = local read "SFDR (dBc)"() -> (w281:dbl[])
        n200 = local read "gain"() -> (w280:dbl[])
        n201 = for {
          tunnel: [w344] -> w286 mode=indexing
          tunnel: w287 -> [w343] mode=indexing
          tunnel: "%5.1f" ("initial string") -> [w342]
          n202 = Format Into String(format string=w342, w343) -> (resulting string=w344:string)  [unwired: 2 in, 1 out]
        }
        n203 = for {
          tunnel: [w335] -> w266 mode=indexing
          tunnel: w280 -> [w334] mode=indexing
          tunnel: w279 -> [w333]
          n204 = Format Into String(format string=w333, w334) -> (resulting string=w335:string)  [unwired: 2 in, 1 out]
        }
        n205 = for {
          tunnel: [w338] -> w265 mode=indexing
          tunnel: w281 -> [w337] mode=indexing
          tunnel: "%5.1f" ("initial string") -> [w336]
          n206 = Format Into String(format string=w336, w337) -> (resulting string=w338:string)  [unwired: 2 in, 1 out]
        }
        n207 = for {
          tunnel: [w341] -> w264 mode=indexing
          tunnel: w283 -> [w340] mode=indexing
          tunnel: "%.3f" ("initial string") -> [w339]
          n208 = Format Into String(format string=w339, w340) -> (resulting string=w341:string)  [unwired: 2 in, 1 out]
        }
        n209 = Build Array(w259, w276, w273, w270, w268, w285, w293, w290, w286, w266, w265, w264) -> (w263:string[][])
        n210 = Transpose 2D Array(2D array=w263) -> (transposed array=w260:string[][])
        "meas table" <- w260
        n211 = flat-sequence {
          tunnel: [w320] -> w261
          tunnel: w260 -> [_]
          tunnel: w257 -> [w318]
          frame #0 {
            n212 = control-ref of="meas table"() -> (w319:refnum<vi>)
            n213 = call "Autosize Columns (Table).vi"("error in (no error)"=w318, "table"=w319) -> ("error out"=w320:errorcluster)  [unwired: 9 in]
          }
        }
      }
      frame "Exit" {
        # "This case is triggered to close the User Interface from framework"
        n214 = Flush Queue(queue=w381, error in (no error)=w383) -> (queue out=w380:refnum<queue>, error out=w379:errorcluster)  [unwired: 1 out]
        n215 = Release Queue(queue=w380, force destroy? (F)=TRUE, error in (no error)=w379) -> (error out=w378:errorcluster)  [unwired: 2 out]
      }
      frame "Handle Error" {
      }
    }
  }
